vi "VCS Get Error Info.vi"(8 "error in (no error)":errorcluster, 11 "errorCodeValue":u32) -> (0 "error out":errorcluster, 3 "errorInfo":string)   [LabVIEW 2019, in "maxonEPOS.lvlib"]
doc: "<B>VCS Get Error Info</B> returns the error information from a received error code."
uses:
  Examples/maxonEPOS.lvlib
  Resources/EposCmd.dll
  Resources/EposCmd64.dll
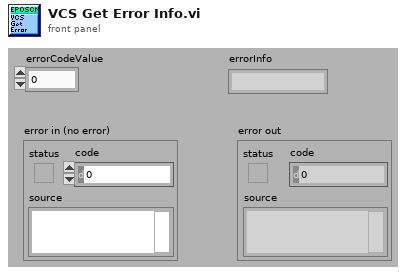
[diagram p1: front panel]
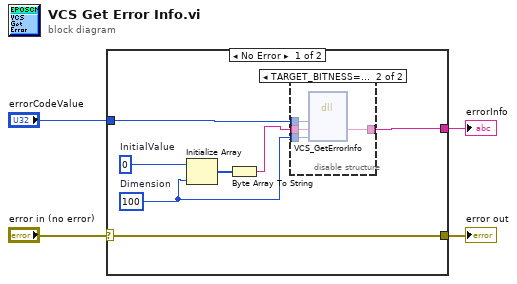
[diagram p0: block diagram]
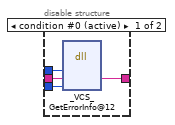
[diagram p2: hidden frame]
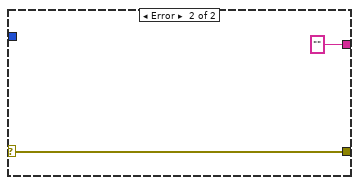
[diagram p3: hidden frame]
diagram:
  n1 = case shown="No Error" "error in (no error)" {
    selector: "error in (no error)" -> [w5 w21]
    tunnel: [w5 w21] -> w3
    tunnel: "errorCodeValue" -> [w11 _]
    tunnel: [w10 "" ("pErrorInfo")] -> w1
    frame No Error {
      w8 = u8 0  # InitialValue
      w6 = 100  # Dimension
      n2 = Initialize Array(w8, w6) -> (w9:u8[])
      n3 = Byte Array To String(unsigned byte array=w9) -> (string=w7:string)
      n4 = disable-structure shown="TARGET_BITNESS==64" {
        disable-tunnel: w11 -> [w15 w19]
        disable-tunnel: [w14 w18] -> w10
        disable-tunnel: w7 -> [w13 w17]
        disable-tunnel: w6 -> [w12 w16]
        frame condition #0 (active) {
          n5 = dll-call lib="C:/workspace/project/scancon/sw/SSI_Tool/InstrumentsInterfaces/Motordriver/maxon EPOS/Resources/EposCmd.*" fn="_VCS_GetErrorInfo@12"("ErrorCodeValue"=w15, "pErrorInfo"=w13, "MaxStrSize"=w12) -> ("pErrorInfo"=w14:string)  [unwired: 6 in, 2 out]
        }
        frame condition #1 {
          n6 = dll-call lib="C:/setup/Resources/EposCmd64.*" fn="VCS_GetErrorInfo" ("EposCmd.dll:_VCS_GetErrorInfo@12")("ErrorCodeValue"=w19, "pErrorInfo"=w17, "MaxStrSize"=w16) -> ("pErrorInfo"=w18:string)  [unwired: 6 in, 2 out]
        }
      }
    }
    frame Error {
    }
  }
  "errorInfo" <- w1
  "error out" <- w3
